vi "M0807 TV Wind.vi"   [LabVIEW 2015]
types:
  T1 = typedef "LVHSConnector.ctl" = refnum<class "BrickReference.lvclass">
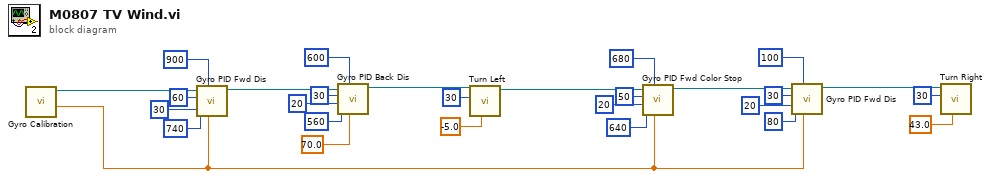
[diagram p0: block diagram]
diagram:
  n1 = call "Gyro Calibration.vi"() -> ("Degrees"=w4:sgl, "NXT/EV3"=w28:T1)  [unwired: 7 in, 1 out]
  n2 = call "Gyro PID Fwd Dis.vi"("Target angle"=w4, "Threshold to stop"=900, "Threshold to slow"=740, "Min. speed"=30, "Max. speed"=60, "EV3 in"=w28) -> ("EV3 out"=w23:T1)  [unwired: 5 in]
  n3 = call "Gyro PID Back Dis.vi"("Target angle"=sgl 70.0, "Threshold to stop"=600, "Threshold to slow"=560, "Min. speed"=20, "Max. speed"=30, "EV3 in"=w23) -> ("EV3 out"=w17:T1)  [unwired: 5 in]
  n4 = call "Turn Left.vi"("Turning angle"=sgl -5.0, "Motor B (right)"=i8 30, "EV3 in"=w17) -> ("EV3 out"=w14:T1)  [unwired: 8 in]
  n5 = call "Gyro PID Fwd Color Stop.vi"("Target angle"=w4, "Threshold to Color"=680 ("Threshold to stop"), "Threshold to slow"=640, "Min. speed"=20, "Max. speed"=50, "EV3 in"=w14) -> ("EV3 out"=w9:T1)  [unwired: 5 in]
  n6 = call "Gyro PID Fwd Dis.vi"("Target angle"=w4, "Threshold to stop"=100, "Threshold to slow"=80, "Min. speed"=20, "Max. speed"=30, "EV3 in"=w9) -> ("EV3 out"=w3:T1)  [unwired: 5 in]
  n7 = call "Turn Right.vi"("Turning angle"=sgl 43.0, "Motor B (right)"=i8 30, "EV3 in"=w3) -> ()  [unwired: 8 in, 1 out]
